vi "Move Impl.vi"(6 "Mode":enum16{"Relative", "Absolute"}(ring), 8 "error in (no error)":errorcluster, 9 "Value (um)":dbl format="%#_13g", 10 "Axis":T1=enum."Y", 11 "Virtual Stage in":refnum<class "Simulated Stage.lvclass">) -> (0 "error out":errorcluster, 3 "Virtual Stage out":refnum<class "Simulated Stage.lvclass">)   [LabVIEW 2023, in "Simulated Stage.lvlib" / "Simulated Stage.lvclass"]
uses:
  Simulated Stage.lvclass
  Stage Controller/Stage Axis.ctl
  Stage Controller/Stage Controller.lvclass
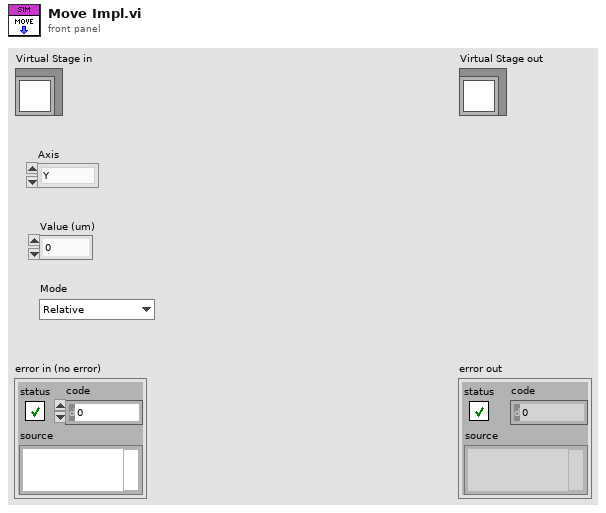
[diagram p1: front panel]
types:
  T1 = typedef "Stage Controller.lvlib/Stage Controller.lvclass/Stage Axis.ctl" = enum16{"unspecified", "X", "Y", "Z"}
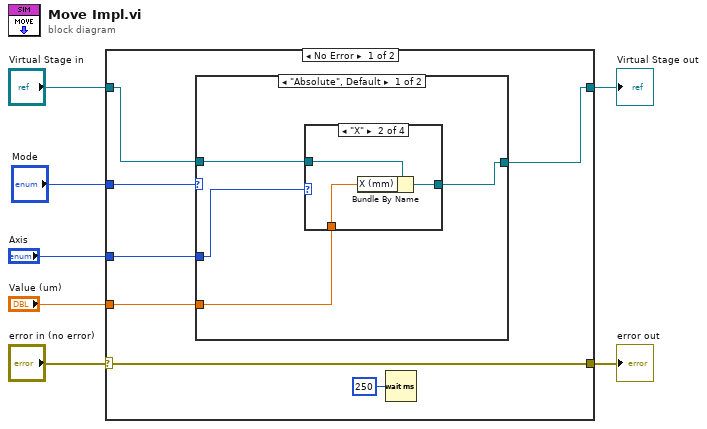
[diagram p0: block diagram]
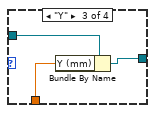
[diagram p3: hidden frame]
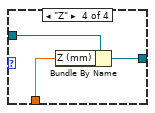
[diagram p4: hidden frame]
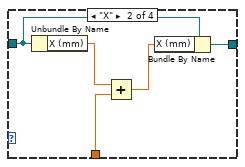
[diagram p6: hidden frame]
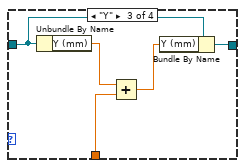
[diagram p7: hidden frame]
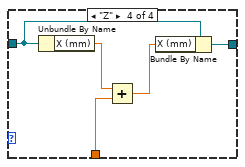
[diagram p8: hidden frame]
diagram:
  n1 = case shown="No Error" "error in (no error)" {
    selector: "error in (no error)" -> [w14 w49]
    tunnel: [w14 w49] -> w6
    tunnel: "Virtual Stage in" -> [w12 w50]
    tunnel: [w11 w50] -> w4
    tunnel: "Mode" -> [w10 _]
    tunnel: "Axis" -> [w13 _]
    tunnel: "Value (um)" -> [w8 _]
    frame No Error {
      n2 = case shown="\"Absolute\", Default" w10 {
        tunnel: w13 -> [w18 w32]
        tunnel: w12 -> [w16 w31]
        tunnel: [w15 w30] -> w11
        tunnel: w8 -> [w17 w29]
        frame "Absolute", Default {
          n3 = case shown="\"X\"" w18 {
            tunnel: w17 -> [_ w20 w24 w26]
            tunnel: w16 -> [w19 w22 w25 w27]
            tunnel: [w19 w21 w23 w28] -> w15
            frame Default {
            }
            frame "X" {
              n4 = Bundle By Name(cluster=w22, "X (mm)"=w20) -> (w21:refnum<class "Simulated Stage.lvclass">)
            }
            frame "Y" {
              n5 = Bundle By Name(cluster=w25, "Y (mm)"=w24) -> (w23:refnum<class "Simulated Stage.lvclass">)
            }
            frame "Z" {
              n6 = Bundle By Name(cluster=w27, "Z (mm)"=w26) -> (w28:refnum<class "Simulated Stage.lvclass">)
            }
          }
        }
        frame "Relative" {
          n7 = case shown="Default" w32 {
            tunnel: w31 -> [w33 w38 w40 w45]
            tunnel: [w33 w37 w41 w46] -> w30
            tunnel: w29 -> [_ w34 w39 w44]
            frame Default {
            }
            frame "X" {
              n8 = Unbundle By Name(w38) -> ("X (mm)"=w36:dbl)
              n9 = Add(x=w36, y=w34) -> (x+y=w35:dbl)
              n10 = Bundle By Name(cluster=w38, "X (mm)"=w35) -> (w37:refnum<class "Simulated Stage.lvclass">)
            }
            frame "Y" {
              n11 = Unbundle By Name(w40) -> ("Y (mm)"=w43:dbl)
              n12 = Add(x=w43, y=w39) -> (x+y=w42:dbl)
              n13 = Bundle By Name(cluster=w40, "Y (mm)"=w42) -> (w41:refnum<class "Simulated Stage.lvclass">)
            }
            frame "Z" {
              n14 = Unbundle By Name(w45) -> ("X (mm)"=w48:dbl)
              n15 = Add(x=w48, y=w44) -> (x+y=w47:dbl)
              n16 = Bundle By Name(cluster=w45, "X (mm)"=w47) -> (w46:refnum<class "Simulated Stage.lvclass">)
            }
          }
        }
      }
      n17 = Wait (ms)(milliseconds to wait=u32 250) -> ()  [unwired: 1 out]
    }
    frame Error {
    }
  }
  "error out" <- w6
  "Virtual Stage out" <- w4
